vi "StopGrab.vi"(1 "error in (no error)":errorcluster, 2 "IGxStream":refnum<k24>, 3 "IGxDevice":refnum<k24>) -> (0 "error out":errorcluster)   [LabVIEW 2013, in "GxLVlib.lvlib"]
uses:
  GxLVlib.lvlib
  C:/Program Files/Daheng Imaging/GalaxySDK/Samples/LabVIEW SDK/x64/GxLVLib/dll/GxIAPINET.dll
  dll/GxIAPINET.dll
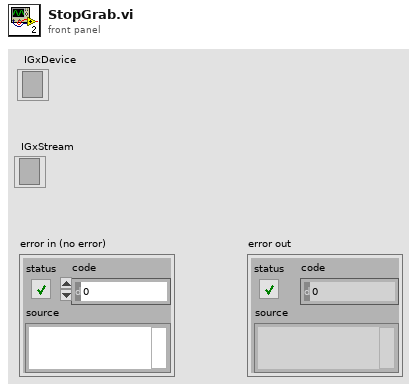
[diagram p1: front panel]
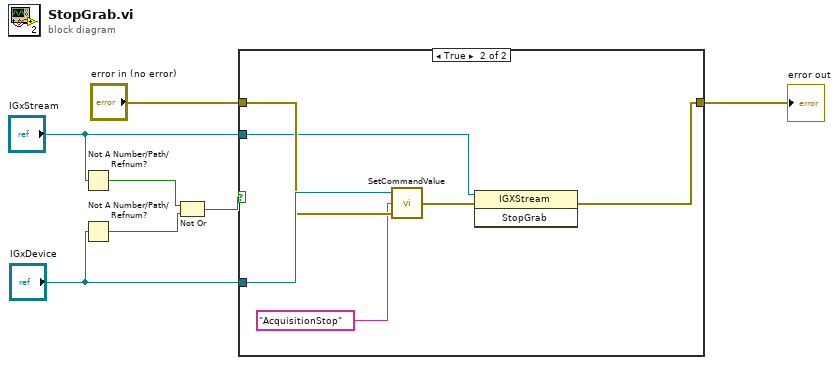
[diagram p0: block diagram]
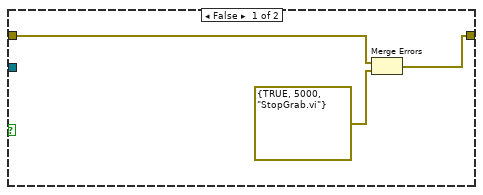
[diagram p2: hidden frame]
diagram:
  n1 = Not A Number/Path/Refnum?(number/path/refnum="IGxStream") -> (NaN/Path/Refnum?=w7:bool)
  n2 = Not A Number/Path/Refnum?(number/path/refnum="IGxDevice") -> (NaN/Path/Refnum?=w6:bool)
  n3 = Not Or(1:w6, 2:w7) -> (0:w5:bool)
  n4 = case shown="True" w5 {
    tunnel: "error in (no error)" -> [w9 w15]
    tunnel: "IGxDevice" -> [_ w16]
    tunnel: "IGxStream" -> [_ w13]
    tunnel: [w8 w11] -> w1
    frame False {
      n5 = Merge Errors(w9, errorcluster {TRUE, 5000, "StopGrab.vi"}) -> (w8:errorcluster)
    }
    frame True {
      n6 = call "SetCommandValue.vi"("error in (no error)"=w15, "Feature Name"="AcquisitionStop", "IGxDevice"=w16) -> ("error out"=w12:errorcluster)
      n7 = invoke class="IGXStream" method="StopGrab"(reference=w13, error in=w12) -> (error out=w11:errorcluster)  [unwired: 1 in, 2 out]
    }
  }
  "error out" <- w1
